vi "Vendor Name.vi"(8 "error in (no error)":errorcluster, 11 "CallVendorRequest in":refnum<class "CallVendorRequest.lvclass">) -> (0 "error out":errorcluster, 2 "Vendor Name":string, 3 "CallVendorRequest out":refnum<class "CallVendorRequest.lvclass">)   [LabVIEW 2022 SP3, in "obs-websocket-lv.lvlib" / "CallVendorRequest.lvclass"]
uses:
  CallVendorRequest.lvclass
  CallVendorRequest.lvclass/CallVendorRequest.ctl
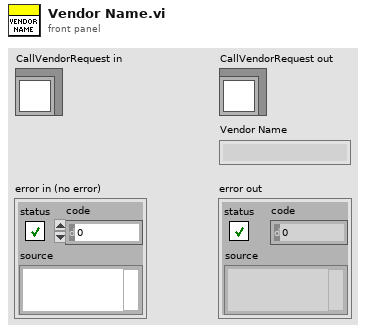
[diagram p1: front panel]
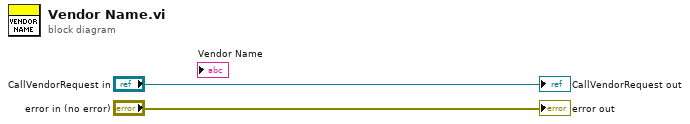
[diagram p0: block diagram]
diagram:
  "error out" <- "error in (no error)"
  "CallVendorRequest out" <- "CallVendorRequest in"
